vi "Get Mouse Position.vi"() -> (1 "X":i32, 2 "Y":i32)   [LabVIEW 2015]
uses:
  USER32.DLL
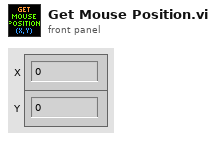
[diagram p1: front panel]
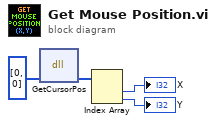
[diagram p0: block diagram]
diagram:
  n1 = dll-call lib="user32.dll" fn="GetCursorPos"("Position"=i32[] [0, 0]) -> ("Position"=w4:i32[])  [unwired: 4 in, 2 out]
  n2 = Index Array(array=w4) -> (element #1=→"X":i32, element #2=→"Y":i32)  [unwired: 2 in]
